vi "Label.vi"(8 "error in (no error)":errorcluster, 10 "Label":T1, 11 "ITX Commands in":refnum<class "ITX Commands.lvclass">) -> (0 "error out":errorcluster, 3 "ITX Commands out":refnum<class "ITX Commands.lvclass">)   [LabVIEW 2016, in "ITX Commands.lvclass"]
uses:
  ITX Commands.lvclass
  ITX Commands.lvclass/ITX Commands.ctl
panel:
  out "resulting string":string
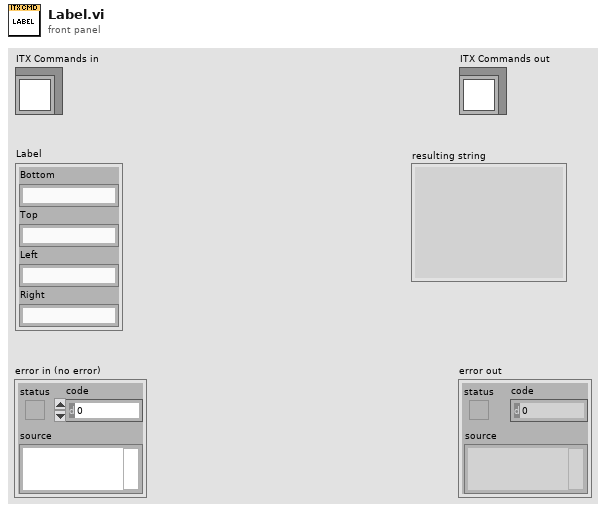
[diagram p1: front panel]
types:
  T1 = cluster{"Bottom":string, "Top":string, "Left":string, "Right":string}
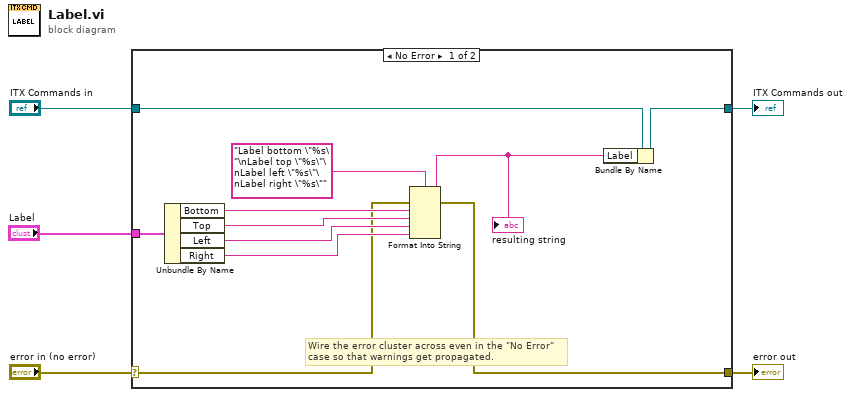
[diagram p0: block diagram]
diagram:
  n1 = case shown="No Error" "error in (no error)" {
    selector: "error in (no error)" -> [w7 w18]
    tunnel: [w6 w18] -> w4
    tunnel: [w9 w17] -> w2
    tunnel: "ITX Commands in" -> [w16 w17]
    tunnel: "Label" -> [w15 _]
    frame No Error {
      # "Wire the error cluster across even in the \"No Error\"\ncase so that warnings get propagated."
      n2 = Unbundle By Name(w15) -> ("Bottom"=w13:string, "Top"=w12:string, "Left"=w11:string, "Right"=w10:string)
      n3 = Format Into String(format string="Label bottom \"%s\"\nLabel top \"%s\"\nLabel left \"%s\"\nLabel right \"%s\"", error in=w7, w13, w12, w11, w10) -> (resulting string=w8:string, error out=w6:errorcluster)  [unwired: 1 in]
      "resulting string" <- w8
      n4 = Bundle By Name(cluster=w16, "Label"=w8) -> (w9:refnum<class "ITX Commands.lvclass">)
    }
    frame Error {
    }
  }
  "error out" <- w4
  "ITX Commands out" <- w2
